vi "Brightness_2011.vi"(3 "Image (Counts)":dbl[][](array[numeric]), 4 "R^2 map":dbl[][](array[numeric]), 5 "Screen&Camera 2":T1={"Screen Orientation"="Regular", "Screen angle"="Flat", "Lens"=enum."FL1-f8x08", "Calibration (mm/pix)"=1.0}) -> (1 "Corrected image":dbl[][](array[numeric]))   [LabVIEW 2013]
uses:
  SubVis/ScreenCam2_TypDEf.ctl
  SubVis/CamAndObj_TypDEf.ctl
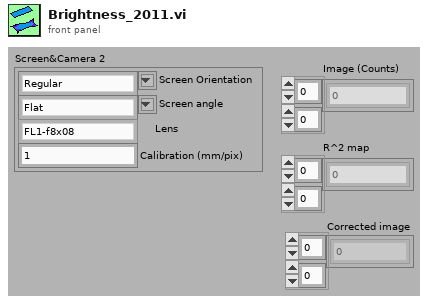
[diagram p1: front panel]
types:
  T1 = typedef "ScreenCam2_TypDEf.ctl" = cluster{"Screen Orientation":string, "Screen angle":string, "Lens":T2, "Calibration (mm/pix)":dbl}
  T2 = typedef "CamAndObj_TypDEf.ctl" = enum16{"FL1-f8x08", "FL1-f8x06", "FL1-f8", "ch300-f50", "FL2G-f8", "FL3M14-f8", "FL3M14-f8x08", "FL3M14-f8x08(2x2)"}
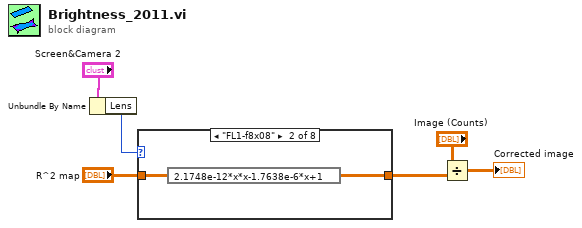
[diagram p0: block diagram]
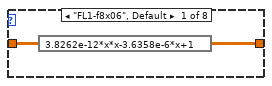
[diagram p2: hidden frame]
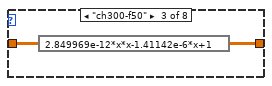
[diagram p3: hidden frame]
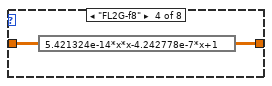
[diagram p4: hidden frame]
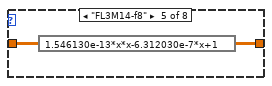
[diagram p5: hidden frame]
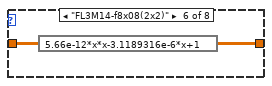
[diagram p6: hidden frame]
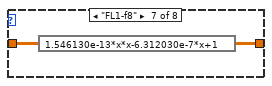
[diagram p7: hidden frame]
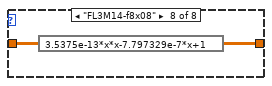
[diagram p8: hidden frame]
diagram:
  n1 = Unbundle By Name("Screen&Camera 2") -> ("Lens"=w4:T2)
  n2 = case shown="\"FL1-f8x08\"" w4 {
    tunnel: "R^2 map" -> [w8 w10 w12 w14 w16 w18 w20 w22]
    tunnel: [w7 w9 w11 w13 w15 w17 w19 w21] -> w2
    frame "FL1-f8x06", Default {
      n3 = expression code="3.8262e-12*x*x-3.6358e-6*x+1"(w8) -> (w7:dbl[][])
    }
    frame "FL1-f8x08" {
      n4 = expression code="2.1748e-12*x*x-1.7638e-6*x+1"(w10) -> (w9:dbl[][])
    }
    frame "ch300-f50" {
      n5 = expression code="2.849969e-12*x*x-1.41142e-6*x+1"(w12) -> (w11:dbl[][])
    }
    frame "FL2G-f8" {
      n6 = expression code="5.421324e-14*x*x-4.242778e-7*x+1"(w14) -> (w13:dbl[][])
    }
    frame "FL3M14-f8" {
      n7 = expression code="1.546130e-13*x*x-6.312030e-7*x+1"(w16) -> (w15:dbl[][])
    }
    frame "FL3M14-f8x08(2x2)" {
      n8 = expression code="5.66e-12*x*x-3.1189316e-6*x+1"(w18) -> (w17:dbl[][])
    }
    frame "FL1-f8" {
      n9 = expression code="1.546130e-13*x*x-6.312030e-7*x+1"(w20) -> (w19:dbl[][])
    }
    frame "FL3M14-f8x08" {
      n10 = expression code="3.5375e-13*x*x-7.797329e-7*x+1"(w22) -> (w21:dbl[][])
    }
  }
  n11 = Divide(x="Image (Counts)", y=w2) -> (x/y=→"Corrected image":dbl[][])
